vi "WS1050_NI6501_Relay_Control_ver1.0.vi"(4 "Ring":u16(ring) items=["All Off", "Bank 1", "Bank 2", "Bank 3"], 10 "Relay_ 11":bool, 11 "error in (no error)":errorcluster, 14 "Relay_ 10":bool) -> (0 "RF_SWitch_Ctrl1":bool=TRUE, 1 "RF_SWitch_Ctrl3":bool=TRUE, 2 "RL_3_SW_PIC":bool, 3 "RF_SWitch_Ctrl6":bool=TRUE, 5 "RF_SWitch_Ctrl2":bool=TRUE, 7 "RL_1_SW_PIC":bool, 9 "RL_2_SW_PIC":bool, 12 "RF_SWitch_Ctrl4":bool=TRUE, 13 "RF_SWitch_Ctrl5":bool=TRUE, 15 "error out":errorcluster)   [LabVIEW 2012]
doc: "I. Description:\nThis example demonstrates how to write values to a digital output channel.\n\nII. Instructions for Running:\n1. Select the digital lines on the DAQ device to be written.\n2. Select a value to write.\nNote: The array control is sized for 8 lines, if using a different amount of lines, change the number of elements in the array to equal the number of lines chosen.\n\nIII. Block Diagram Steps:\n1. Create a Digital Output channel. Use one channel for all lines. You can alternatively use one channel for each line, but then use a different polymorphic version of the DAQmx Write VI.\n2. Call the Start VI to start the task.\n3. Write the digital Boolean array data in a loop until the user hits the stop button or an error occurs. This write VI writes a single sample of digital data on demand, so no timeout is necessary.\n4. Call the Clear Task VI to clear the Task.\n5. Use the popup dialog box to display an error or warning if any.\n\nIV. I/O Connections Overview:\nMake sure your signal output terminals match the Lines I/O Control. In this case wire the item to receive the signal to the first eight digital lines on your DAQ Device."
uses:
  <vilib>/DAQmx/write.llb/DAQmx Write (Digital Bool 1Line 1Point).vi
  <vilib>/DAQmx/create/channels.llb/DAQmx Create Channel (DO-Digital Output).vi
  <vilib>/DAQmx/miscellaneous.llb/DAQmx Fill In Error Info.vi
panel:
  in  "Lines 11":tag="Dev2/port0/line1" caption="Lines"
  in  "Lines 10":tag="Dev2/port1/line2" caption="Lines"
  in  "Lines 9":tag="Dev2/port1/line4" caption="Lines"
  in  "Lines 8":tag="Dev2/port2/line7" caption="Lines"
  in  "Lines 7":tag="Dev2/port2/line6" caption="Lines"
  in  "Lines 6":tag="Dev2/port2/line5" caption="Lines"
  in  "Lines 5":tag="Dev2/port2/line4" caption="Lines"
  in  "Lines 4":tag="Dev2/port2/line3" caption="Lines"
  in  "Lines 3":tag="Dev2/port2/line2" caption="Lines"
  in  "Lines 2":tag="Dev2/port2/line1" caption="Lines"
  in  "Lines":tag="Dev2/port2/line0"
  # "For instructions, select Help>>Show Context Help"
  # "Channel Parameters"
  # "Pin 11"
  # "Pin 14"
  # "Pin16"
  # "Line 5"
  # "Line 2"
  # "Line 0"
  # "Pin 09"
  # "Pin 13"
  # "Pin 15"
  # "Line 7"
  # "Line 3"
  # "Line 1"
  # "Pin 6"
  # "Pin 10"
  # "Pin 12"
  # "Line 4 Port1"
  # "Line 6"
  # "Line 4"
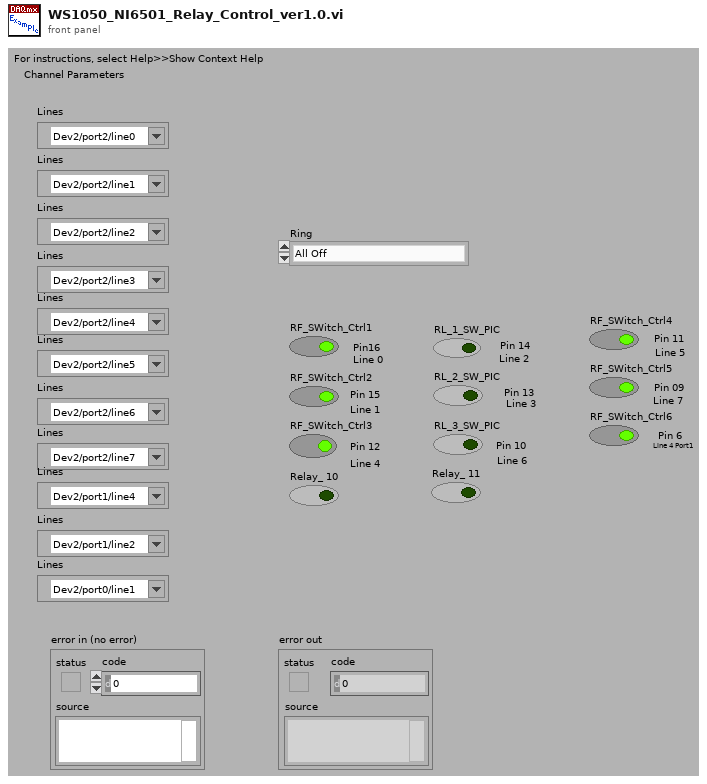
[diagram p1: front panel]
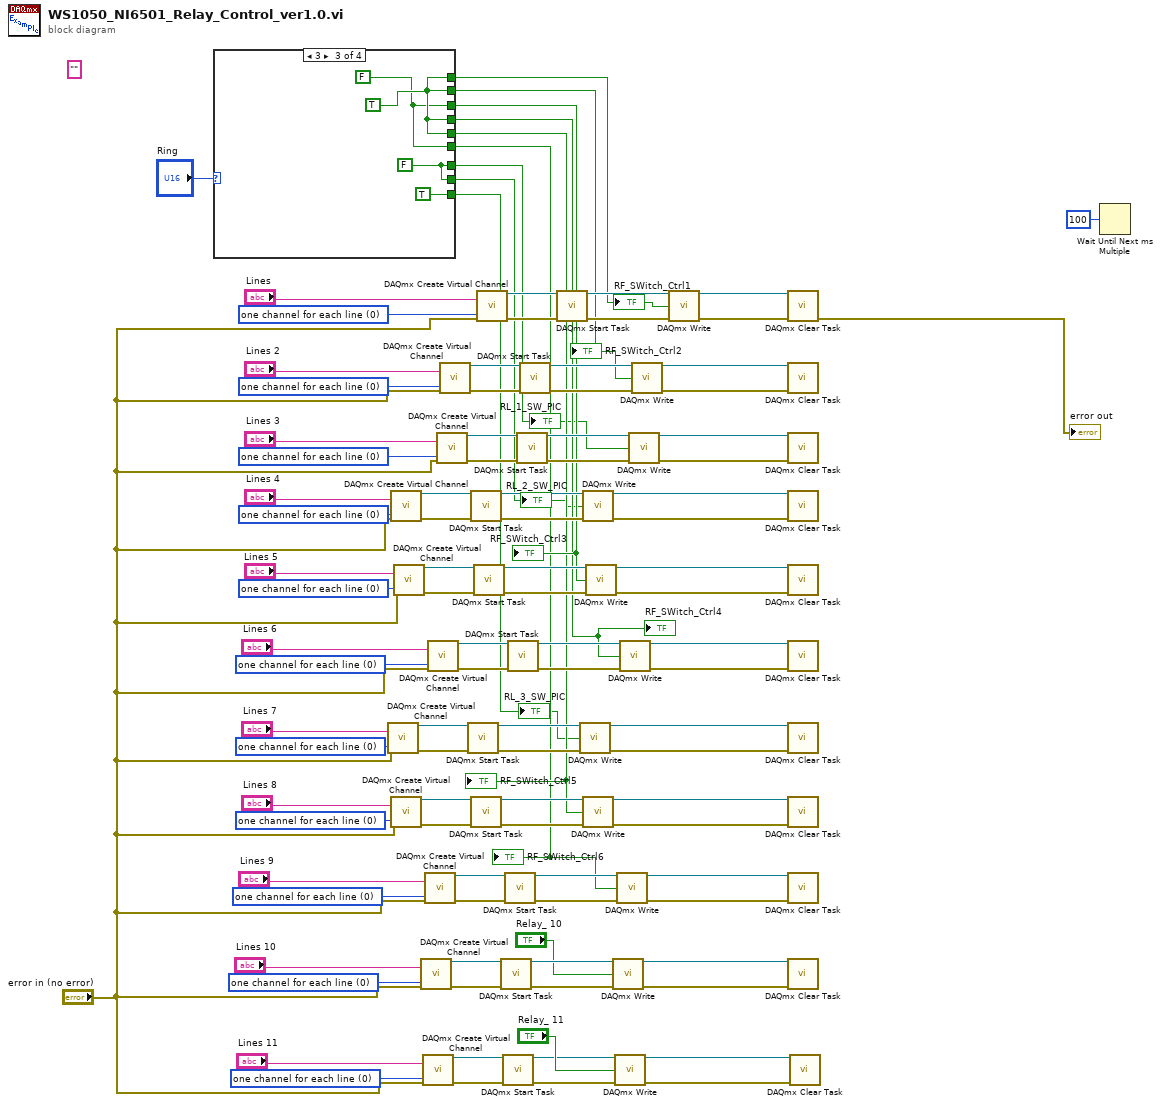
[diagram p0: block diagram]
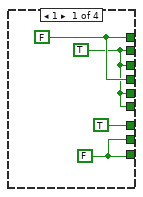
[diagram p2: hidden frame]
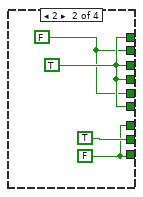
[diagram p3: hidden frame]
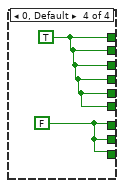
[diagram p4: hidden frame]
diagram:
  w2 = 0 items=["one channel for each line", "one channel for all lines"] ("line grouping")
  (unwired) ""
  w30 = 0 items=["one channel for each line", "one channel for all lines"] ("line grouping")
  w31 = 0 items=["one channel for each line", "one channel for all lines"] ("line grouping")
  w46 = 0 items=["one channel for each line", "one channel for all lines"] ("line grouping")
  w47 = 0 items=["one channel for each line", "one channel for all lines"] ("line grouping")
  w78 = 0 items=["one channel for each line", "one channel for all lines"] ("line grouping")
  w63 = 0 items=["one channel for each line", "one channel for all lines"] ("line grouping")
  w62 = 0 items=["one channel for each line", "one channel for all lines"] ("line grouping")
  w79 = 0 items=["one channel for each line", "one channel for all lines"] ("line grouping")
  w94 = 0 items=["one channel for each line", "one channel for all lines"] ("line grouping")
  w96 = 0 items=["one channel for each line", "one channel for all lines"] ("line grouping")
  n1 = case shown="3" "Ring" {
    tunnel: [w107 w111 w113 w117] -> w21
    tunnel: [w106 w110 w113 w117] -> w20
    tunnel: [w106 w111 w112 w117] -> w19
    tunnel: [w107 w111 w113 w117] -> w18
    tunnel: [w106 w110 w113 w117] -> w17
    tunnel: [w106 w111 w112 w117] -> w16
    tunnel: [TRUE ("RF_SWitch_Ctrl1") w108 w115 w116] -> w15
    tunnel: [w104 TRUE ("RF_SWitch_Ctrl1") w115 w116] -> w14
    tunnel: [w104 w108 TRUE ("RF_SWitch_Ctrl1") w116] -> w13
    frame 1 {
      w104 = FALSE ("RF_SWitch_Ctrl1")
      w106 = TRUE ("RF_SWitch_Ctrl1")
      w107 = FALSE ("RF_SWitch_Ctrl1")
    }
    frame 2 {
      w108 = FALSE ("RF_SWitch_Ctrl1")
      w111 = TRUE ("RF_SWitch_Ctrl1")
      w110 = FALSE ("RF_SWitch_Ctrl1")
    }
    frame 3 {
      w115 = FALSE ("RF_SWitch_Ctrl1")
      w113 = TRUE ("RF_SWitch_Ctrl1")
      w112 = FALSE ("RF_SWitch_Ctrl1")
    }
    frame 0, Default {
      w117 = TRUE ("RF_SWitch_Ctrl1")
      w116 = FALSE ("RF_SWitch_Ctrl1")
    }
  }
  "RF_SWitch_Ctrl1" <- w21
  "RF_SWitch_Ctrl2" <- w20
  "RL_1_SW_PIC" <- w15
  "RF_SWitch_Ctrl3" <- w19
  "RL_2_SW_PIC" <- w14
  "RF_SWitch_Ctrl4" <- w18
  "RF_SWitch_Ctrl5" <- w17
  "RL_3_SW_PIC" <- w13
  "RF_SWitch_Ctrl6" <- w16
  n2 = call-poly <vilib>:"DAQmx Create Virtual Channel.vi"("lines"="Lines 7", "line grouping"=w31, "error in"="error in (no error)") -> ("task out"=w34:refnum<k21>, "error out"=w33:errorcluster)  [unwired: 11 in]
  n3 = call-poly <vilib>:"DAQmx Create Virtual Channel.vi"("lines"="Lines 4", "line grouping"=w78, "error in"="error in (no error)") -> ("task out"=w75:refnum<k21>, "error out"=w76:errorcluster)  [unwired: 11 in]
  n4 = call-poly <vilib>:"DAQmx Create Virtual Channel.vi"("lines"="Lines 8", "line grouping"=w46, "error in"="error in (no error)") -> ("task out"=w43:refnum<k21>, "error out"=w44:errorcluster)  [unwired: 11 in]
  n5 = call-poly <vilib>:"DAQmx Create Virtual Channel.vi"("lines"="Lines 5", "line grouping"=w63, "error in"="error in (no error)") -> ("task out"=w66:refnum<k21>, "error out"=w65:errorcluster)  [unwired: 11 in]
  n6 = call-poly <vilib>:"DAQmx Create Virtual Channel.vi"("lines"="Lines 10", "line grouping"=w30, "error in"="error in (no error)") -> ("task out"=w27:refnum<k21>, "error out"=w28:errorcluster)  [unwired: 11 in]
  n7 = call-poly <vilib>:"DAQmx Create Virtual Channel.vi"("lines"="Lines 11", "line grouping"=w2, "error in"="error in (no error)") -> ("task out"=w5:refnum<k21>, "error out"=w4:errorcluster)  [unwired: 11 in]
  n8 = call-poly <vilib>:"DAQmx Create Virtual Channel.vi"("lines"="Lines 9", "line grouping"=w47, "error in"="error in (no error)") -> ("task out"=w50:refnum<k21>, "error out"=w49:errorcluster)  [unwired: 11 in]
  n9 = call-poly <vilib>:"DAQmx Create Virtual Channel.vi"("lines"="Lines 6", "line grouping"=w62, "error in"="error in (no error)") -> ("task out"=w59:refnum<k21>, "error out"=w60:errorcluster)  [unwired: 11 in]
  n10 = call-poly <vilib>:"DAQmx Create Virtual Channel.vi"("lines"="Lines 3", "line grouping"=w79, "error in"="error in (no error)") -> ("task out"=w82:refnum<k21>, "error out"=w81:errorcluster)  [unwired: 11 in]
  n11 = call-poly <vilib>:"DAQmx Create Virtual Channel.vi"("lines"="Lines 2", "line grouping"=w94, "error in"="error in (no error)") -> ("task out"=w91:refnum<k21>, "error out"=w92:errorcluster)  [unwired: 11 in]
  n12 = call <vilib>:"DAQmx Start Task.vi"("task/channels in"=w34, "error in"=w33) -> ("task out"=w36:refnum<k21>, "error out"=w38:errorcluster)  [unwired: 12 in]
  n13 = call <vilib>:"DAQmx Start Task.vi"("task/channels in"=w75, "error in"=w76) -> ("task out"=w73:refnum<k21>, "error out"=w71:errorcluster)  [unwired: 12 in]
  n14 = call <vilib>:"DAQmx Start Task.vi"("task/channels in"=w43, "error in"=w44) -> ("task out"=w41:refnum<k21>, "error out"=w39:errorcluster)  [unwired: 12 in]
  n15 = call <vilib>:"DAQmx Start Task.vi"("task/channels in"=w66, "error in"=w65) -> ("task out"=w68:refnum<k21>, "error out"=w70:errorcluster)  [unwired: 12 in]
  n16 = call-poly <vilib>:"DAQmx Create Virtual Channel.vi"("lines"="Lines", "line grouping"=w96, "error in"="error in (no error)") -> ("task out"=w99:refnum<k21>, "error out"=w98:errorcluster)  [unwired: 11 in]
  n17 = call <vilib>:"DAQmx Start Task.vi"("task/channels in"=w27, "error in"=w28) -> ("task out"=w25:refnum<k21>, "error out"=w23:errorcluster)  [unwired: 12 in]
  n18 = call <vilib>:"DAQmx Start Task.vi"("task/channels in"=w5, "error in"=w4) -> ("task out"=w7:refnum<k21>, "error out"=w9:errorcluster)  [unwired: 12 in]
  n19 = call <vilib>:"DAQmx Start Task.vi"("task/channels in"=w50, "error in"=w49) -> ("task out"=w52:refnum<k21>, "error out"=w54:errorcluster)  [unwired: 12 in]
  n20 = call <vilib>:"DAQmx Start Task.vi"("task/channels in"=w59, "error in"=w60) -> ("task out"=w57:refnum<k21>, "error out"=w55:errorcluster)  [unwired: 12 in]
  n21 = call <vilib>:"DAQmx Start Task.vi"("task/channels in"=w82, "error in"=w81) -> ("task out"=w84:refnum<k21>, "error out"=w86:errorcluster)  [unwired: 12 in]
  n22 = call <vilib>:"DAQmx Start Task.vi"("task/channels in"=w91, "error in"=w92) -> ("task out"=w89:refnum<k21>, "error out"=w87:errorcluster)  [unwired: 12 in]
  n23 = call <vilib>:"DAQmx Start Task.vi"("task/channels in"=w99, "error in"=w98) -> ("task out"=w101:refnum<k21>, "error out"=w103:errorcluster)  [unwired: 12 in]
  n24 = call-poly <vilib>:"DAQmx Write.vi"("task/channels in"=w36, "data"=w13, "error in"=w38) -> ("task out"=w35:refnum<k21>, "error out"=w37:errorcluster)  [unwired: 10 in, 1 out]
  n25 = call-poly <vilib>:"DAQmx Write.vi"("task/channels in"=w73, "data"=w14, "error in"=w71) -> ("task out"=w74:refnum<k21>, "error out"=w72:errorcluster)  [unwired: 10 in, 1 out]
  n26 = call-poly <vilib>:"DAQmx Write.vi"("task/channels in"=w41, "data"=w17, "error in"=w39) -> ("task out"=w42:refnum<k21>, "error out"=w40:errorcluster)  [unwired: 10 in, 1 out]
  n27 = call-poly <vilib>:"DAQmx Write.vi"("task/channels in"=w68, "data"=w19, "error in"=w70) -> ("task out"=w67:refnum<k21>, "error out"=w69:errorcluster)  [unwired: 10 in, 1 out]
  n28 = call-poly <vilib>:"DAQmx Write.vi"("task/channels in"=w25, "data"="Relay_ 10", "error in"=w23) -> ("task out"=w26:refnum<k21>, "error out"=w24:errorcluster)  [unwired: 10 in, 1 out]
  n29 = call-poly <vilib>:"DAQmx Write.vi"("task/channels in"=w7, "data"="Relay_ 11", "error in"=w9) -> ("task out"=w6:refnum<k21>, "error out"=w8:errorcluster)  [unwired: 10 in, 1 out]
  n30 = call-poly <vilib>:"DAQmx Write.vi"("task/channels in"=w52, "data"=w16, "error in"=w54) -> ("task out"=w51:refnum<k21>, "error out"=w53:errorcluster)  [unwired: 10 in, 1 out]
  n31 = call-poly <vilib>:"DAQmx Write.vi"("task/channels in"=w57, "data"=w18, "error in"=w55) -> ("task out"=w58:refnum<k21>, "error out"=w56:errorcluster)  [unwired: 10 in, 1 out]
  n32 = call-poly <vilib>:"DAQmx Write.vi"("task/channels in"=w84, "data"=w15, "error in"=w86) -> ("task out"=w83:refnum<k21>, "error out"=w85:errorcluster)  [unwired: 10 in, 1 out]
  n33 = call-poly <vilib>:"DAQmx Write.vi"("task/channels in"=w89, "data"=w20, "error in"=w87) -> ("task out"=w90:refnum<k21>, "error out"=w88:errorcluster)  [unwired: 10 in, 1 out]
  n34 = call-poly <vilib>:"DAQmx Write.vi"("task/channels in"=w101, "data"=w21, "error in"=w103) -> ("task out"=w100:refnum<k21>, "error out"=w102:errorcluster)  [unwired: 10 in, 1 out]
  n35 = call <vilib>:"DAQmx Clear Task.vi"("task in"=w100, "error in"=w102) -> ("error out"=→"error out":errorcluster)  [unwired: 13 in]
  n36 = call <vilib>:"DAQmx Clear Task.vi"("task in"=w90, "error in"=w88) -> ()  [unwired: 13 in, 1 out]
  n37 = call <vilib>:"DAQmx Clear Task.vi"("task in"=w83, "error in"=w85) -> ()  [unwired: 13 in, 1 out]
  n38 = call <vilib>:"DAQmx Clear Task.vi"("task in"=w74, "error in"=w72) -> ()  [unwired: 13 in, 1 out]
  n39 = call <vilib>:"DAQmx Clear Task.vi"("task in"=w67, "error in"=w69) -> ()  [unwired: 13 in, 1 out]
  n40 = call <vilib>:"DAQmx Clear Task.vi"("task in"=w58, "error in"=w56) -> ()  [unwired: 13 in, 1 out]
  n41 = call <vilib>:"DAQmx Clear Task.vi"("task in"=w35, "error in"=w37) -> ()  [unwired: 13 in, 1 out]
  n42 = call <vilib>:"DAQmx Clear Task.vi"("task in"=w42, "error in"=w40) -> ()  [unwired: 13 in, 1 out]
  n43 = call <vilib>:"DAQmx Clear Task.vi"("task in"=w51, "error in"=w53) -> ()  [unwired: 13 in, 1 out]
  n44 = call <vilib>:"DAQmx Clear Task.vi"("task in"=w26, "error in"=w24) -> ()  [unwired: 13 in, 1 out]
  n45 = call <vilib>:"DAQmx Clear Task.vi"("task in"=w6, "error in"=w8) -> ()  [unwired: 13 in, 1 out]
  n46 = Wait Until Next ms Multiple(millisecond multiple=u32 100 ("milliseconds to wait")) -> ()  [unwired: 1 out]
